vi "Calc Distance Matrix.vi"(8 "error in (no error)":errorcluster, 11 "TSP Class in":refnum<class "TSP Class.lvclass">) -> (0 "error out":errorcluster, 3 "TSP Class out":refnum<class "TSP Class.lvclass">)   [LabVIEW 2015, in "TSP Library.lvlib" / "TSP Class.lvclass"]
uses:
  TSP Class.lvclass
  TSP Class.lvclass/TSP Class.ctl
  TSP Library.lvlib
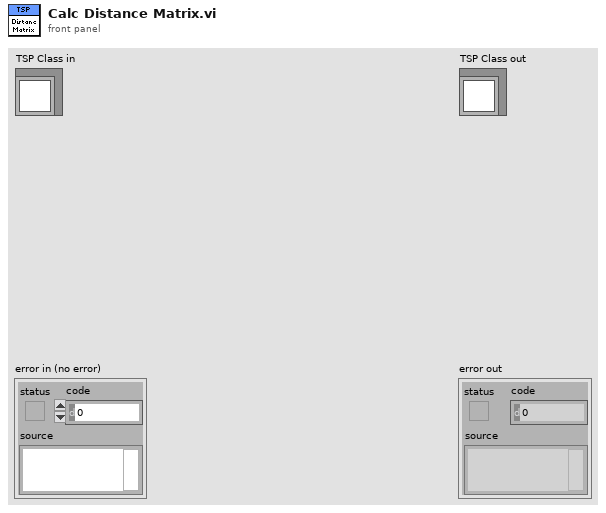
[diagram p1: front panel]
types:
  T1 = typedef "TSP Library.lvlib/Coordinate.ctl" = cluster{"x":dbl, "y":dbl}
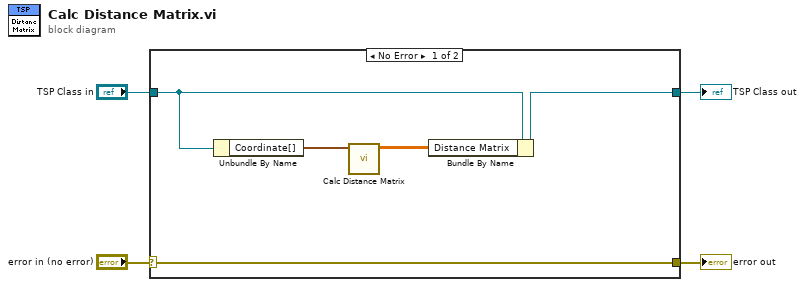
[diagram p0: block diagram]
diagram:
  n1 = case shown="No Error" "error in (no error)" {
    selector: "error in (no error)" -> [w9 w11]
    tunnel: [w9 w11] -> w3
    tunnel: [w7 w10] -> w1
    tunnel: "TSP Class in" -> [w8 w10]
    frame No Error {
      n2 = Unbundle By Name(w8) -> ("Coordinate[]"=w6:T1[])
      n3 = call "Calc Distance Matrix.vi"("Coordinate[]"=w6) -> ("Distance Matrix"=w5:dbl[][])  [unwired: 10 in]
      n4 = Bundle By Name(cluster=w8, "Distance Matrix"=w5) -> (w7:refnum<class "TSP Class.lvclass">)
    }
    frame Error {
    }
  }
  "error out" <- w3
  "TSP Class out" <- w1
